vi "Dashboard Main.vi"() -> ()   [LabVIEW 2012]
uses:
  <vilib>/event_ctls.llb/eventvkey.ctl
  <vilib>/Utility/config.llb/Read Key (String).vi
  <vilib>/Utility/config.llb/Read Key (I32).vi
  <vilib>/Utility/config.llb/Write Key (String).vi
  <vilib>/Utility/config.llb/Write Key (I32).vi
  <vilib>/Utility/config.llb/NI_LVConfig.lvlib
panel:
  out "Battery Value":dbl(slide) scale=0.0..14.0 scale format="%#_2e"
  out "Battery":sgl(graph)
  in  "Camera Settings":T1={"Frate Rate"=30, "Compression"=30, "Size"=0} {"Frate Rate" scale=1.0..30.0; "Size" items=["640x480", "320x240", "160x120"]}
  out "Mode":T2(ring)=enum.""
  out "Camera IP":string="10.16.76.11"
  out "JS1 Z":dbl(slide) scale=-1.0..1.0 scale format="%#_2e"
  out "JS2 Z":dbl(slide) scale=-1.0..1.0 scale format="%#_2e"
  out "Joystick 1":cluster{"X":dbl, "Y":dbl}[](graph)
  out "Joystick 2":cluster{"X":dbl, "Y":dbl}[](graph)
  out "JS Buttons 1":T3
  out "JS Buttons 2":T3
  out "MotorSlide4":dbl(slide) scale=-1.0..1.0 scale format="%#_2e"
  out "MotorSlide3":dbl(slide) scale=-1.0..1.0 scale format="%#_2e"
  out "MotorSlide2":dbl(slide) scale=-1.0..1.0 scale format="%#_2e"
  in  "MotorName3":string="Front Left"
  in  "MotorName4":string="Front Right"
  in  "MotorName1":string="Rear Left"
  in  "MotorName2":string="Rear Right"
  out "MotorChart4":dbl(graph)
  out "MotorChart3":dbl(graph)
  out "MotorChart2":dbl(graph)
  out "MotorSlide1":dbl(slide) scale=-1.0..1.0 scale format="%#_2e"
  out "MotorChart1":dbl(graph)
  out "Robot IP":string="0.0.0.0"
  in  "Dashboard Tab":enum32{"Operation", "Test", "Checklist"}(tab)
  in  "Checkbox 2":bool
  in  "Checkbox 1":bool
  in  "Slider 1":dbl(slide) scale=0.0..100.0
  in  "Slider":dbl(slide) scale=0.0..100.0 scale format="%#_3g"
  in  "On/Off":bool caption="Solenoid"
  in  "Test Name":u16(ring) items=["Select the test to run...", "Example Test", "-------------------------------", "List of tests is built in robot code.", "Replace with your own automated tests."]
  in  "Test Tree":string(tree)
  in  "Motor":cluster{"Value":dbl, "Enable":bool} {"Value" scale=-1.0..1.0 scale format="%#_3g"}
  out "Progress":T4 {"Test Progress" scale=0.0..100.0}
  in  "Rev/Fwd":cluster{"Forward":bool, "Reverse":bool}
  in  "Ring":u16(ring) items=["Auto", "Fixed indoor", "Fixed outdoor 1", "Fixed outdoor 2", "Fixed fluorescent 1", "Fixed fluorescent 2", "Hold current"]
  in  "Listbox":i32(listbox)
  in  "Viewer":T5(tab)
  out "Mbps":dbl format="%#.1g"
  in  "Enable":bool=TRUE
  in  "DB Camera Config":bool
  out "Mbps":bool
  out "fps":dbl format="%#.1g"
  out "Image Error Message":string="Timeout in Camera Communications"
  out "Camera Image":T6(plugin-control)
  out "Buttons 1":cluster{"1":bool, "2":bool, "3":bool}
  out "Kinect 1":cluster{"X":dbl, "Y":dbl, "Z":dbl} {"X" scale=1.0..-1.0; "Y" scale=1.0..-1.0; "Z" scale=1.0..-1.0}
  out "Buttons 2":cluster{"1":bool, "2":bool, "3":bool}
  out "Kinect 2":cluster{"X":dbl, "Y":dbl, "Z":dbl} {"X" scale=1.0..-1.0; "Y" scale=1.0..-1.0; "Z" scale=1.0..-1.0}
  out "Version":string
  out "Skeleton Picture":picture
  out "Players":i8
  out "Tree":string(tree)
  # "Drive & Motors"
  # "Robot IP:"
  # "Customize by placing controls and indicators here and name to match\nDashboard Variables on robot."
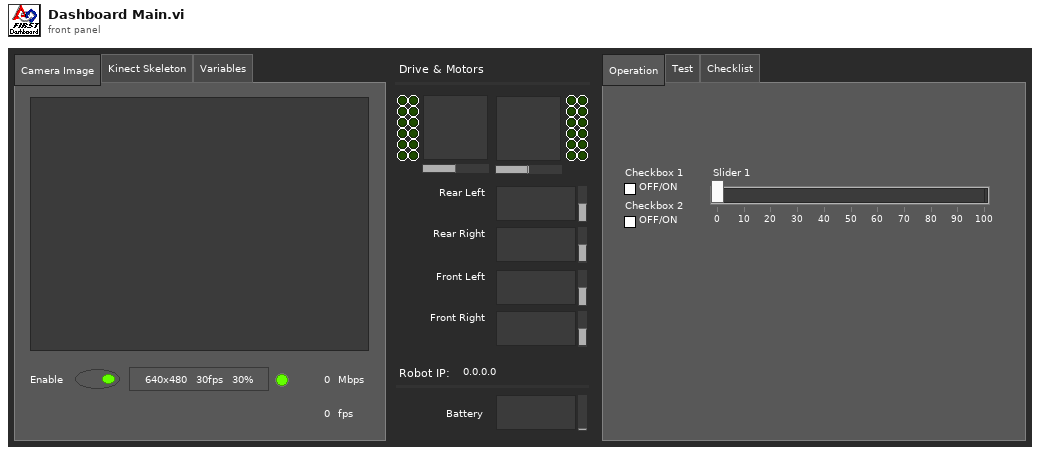
[diagram p1: front panel]
types:
  T1 = cluster{"Frate Rate":i32, "Compression":i32, "Size":u16}
  T2 = enum8{"Tele-Op Disabled", "Tele-Op Enabled", "Auto Disabled", "Auto Enabled", "Test Disabled", "Test Enabled", ""}
  T3 = cluster{bool, bool, bool, bool, bool, bool, bool, bool, bool, bool, bool, bool}
  T4 = cluster{"Test Progress":u8, "Test Progress Text":string}
  T5 = enum32{"Camera Image", "Kinect Skeleton", "Variables"}
  T6 = typedef "IMAQ Image.ctl" = refnum<image>
  T7 = typedef "Image Type" = u32
  T8 = cluster{"Competition mode":bool, "Robot Link":bool, "Autonomous":bool, "Enabled":bool, "E-Stop":bool, "Simulated":bool, "TestMode":bool, "Docked Window":bool}
  T9 = cluster{"Boolean Array[0]":bool, "Boolean Array[1]":bool, "Boolean Array[2]":bool, "Boolean Array[3]":bool, "Boolean Array[4]":bool, "Boolean Array[5]":bool, "Boolean Array[6]":bool, "Boolean Array[7]":bool, "Boolean Array[8]":bool, "Boolean Array[9]":bool, "Boolean Array[10]":bool, "Boolean Array[11]":bool}
  T10 = typedef "LVBoundsTypeDef.ctl" = cluster{"Width":u32, "Height":u32}
  T11 = typedef "SkeletonTrackState.ctl" = enum32{"NotTracked", "PositionOnly", "Tracked"}
  T12 = cluster{"TrackingState":u8[], "Position":cluster{"x":sgl, "y":sgl, "z":sgl}, cluster{"x":sgl, "y":sgl, "z":sgl, sgl}[], "TrackState":T11}
  T13 = cluster{cluster{"ScaledToPercentRange":dbl, "ScaledToPercentRange":dbl, "ScaledToPercentRange":dbl}, cluster{bool, bool, bool}}[]
  T14 = cluster{cluster{"ScaledToPercentRange":dbl, "ScaledToPercentRange":dbl, "ScaledToPercentRange":dbl}, cluster{bool, bool, bool}}
  T15 = cluster{"ScaledToPercentRange":dbl, "ScaledToPercentRange":dbl, "ScaledToPercentRange":dbl}
  T16 = typedef "LVRectTypeDef.ctl" = cluster{"Left":i16, "Top":i16, "Right":i16, "Bottom":i16}
  T17 = typedef "NI_LVConfig.lvlib/Config Data RefNum.ctl" = refnum<k1>
  T18 = typedef "eventvkey.ctl" = enum16{"ASCII", "Enter", "Return", "Shift", "Ctrl", "Alt", "Cmd", "Opt", "Caps", "NumLock", "Clear", "Break", "Up", "Down", "Left", "Right", "Insert", "Delete", "Home", "End", "PageUp", "PageDown", "Escape", "Help", "Pause", "ScrollLock", "F1", "F2", "F3", "F4", "F5", "F6", "F7", "F8", "F9", "F10", "F11", "F12", "F13", "F14", "F15", "F16", "F17", "F18", "F19", "F20", "F21", "F22", "F23", "F24", "Play", "VolumeUp", "VolumeDown", "Mute", "Two Byte Char"}
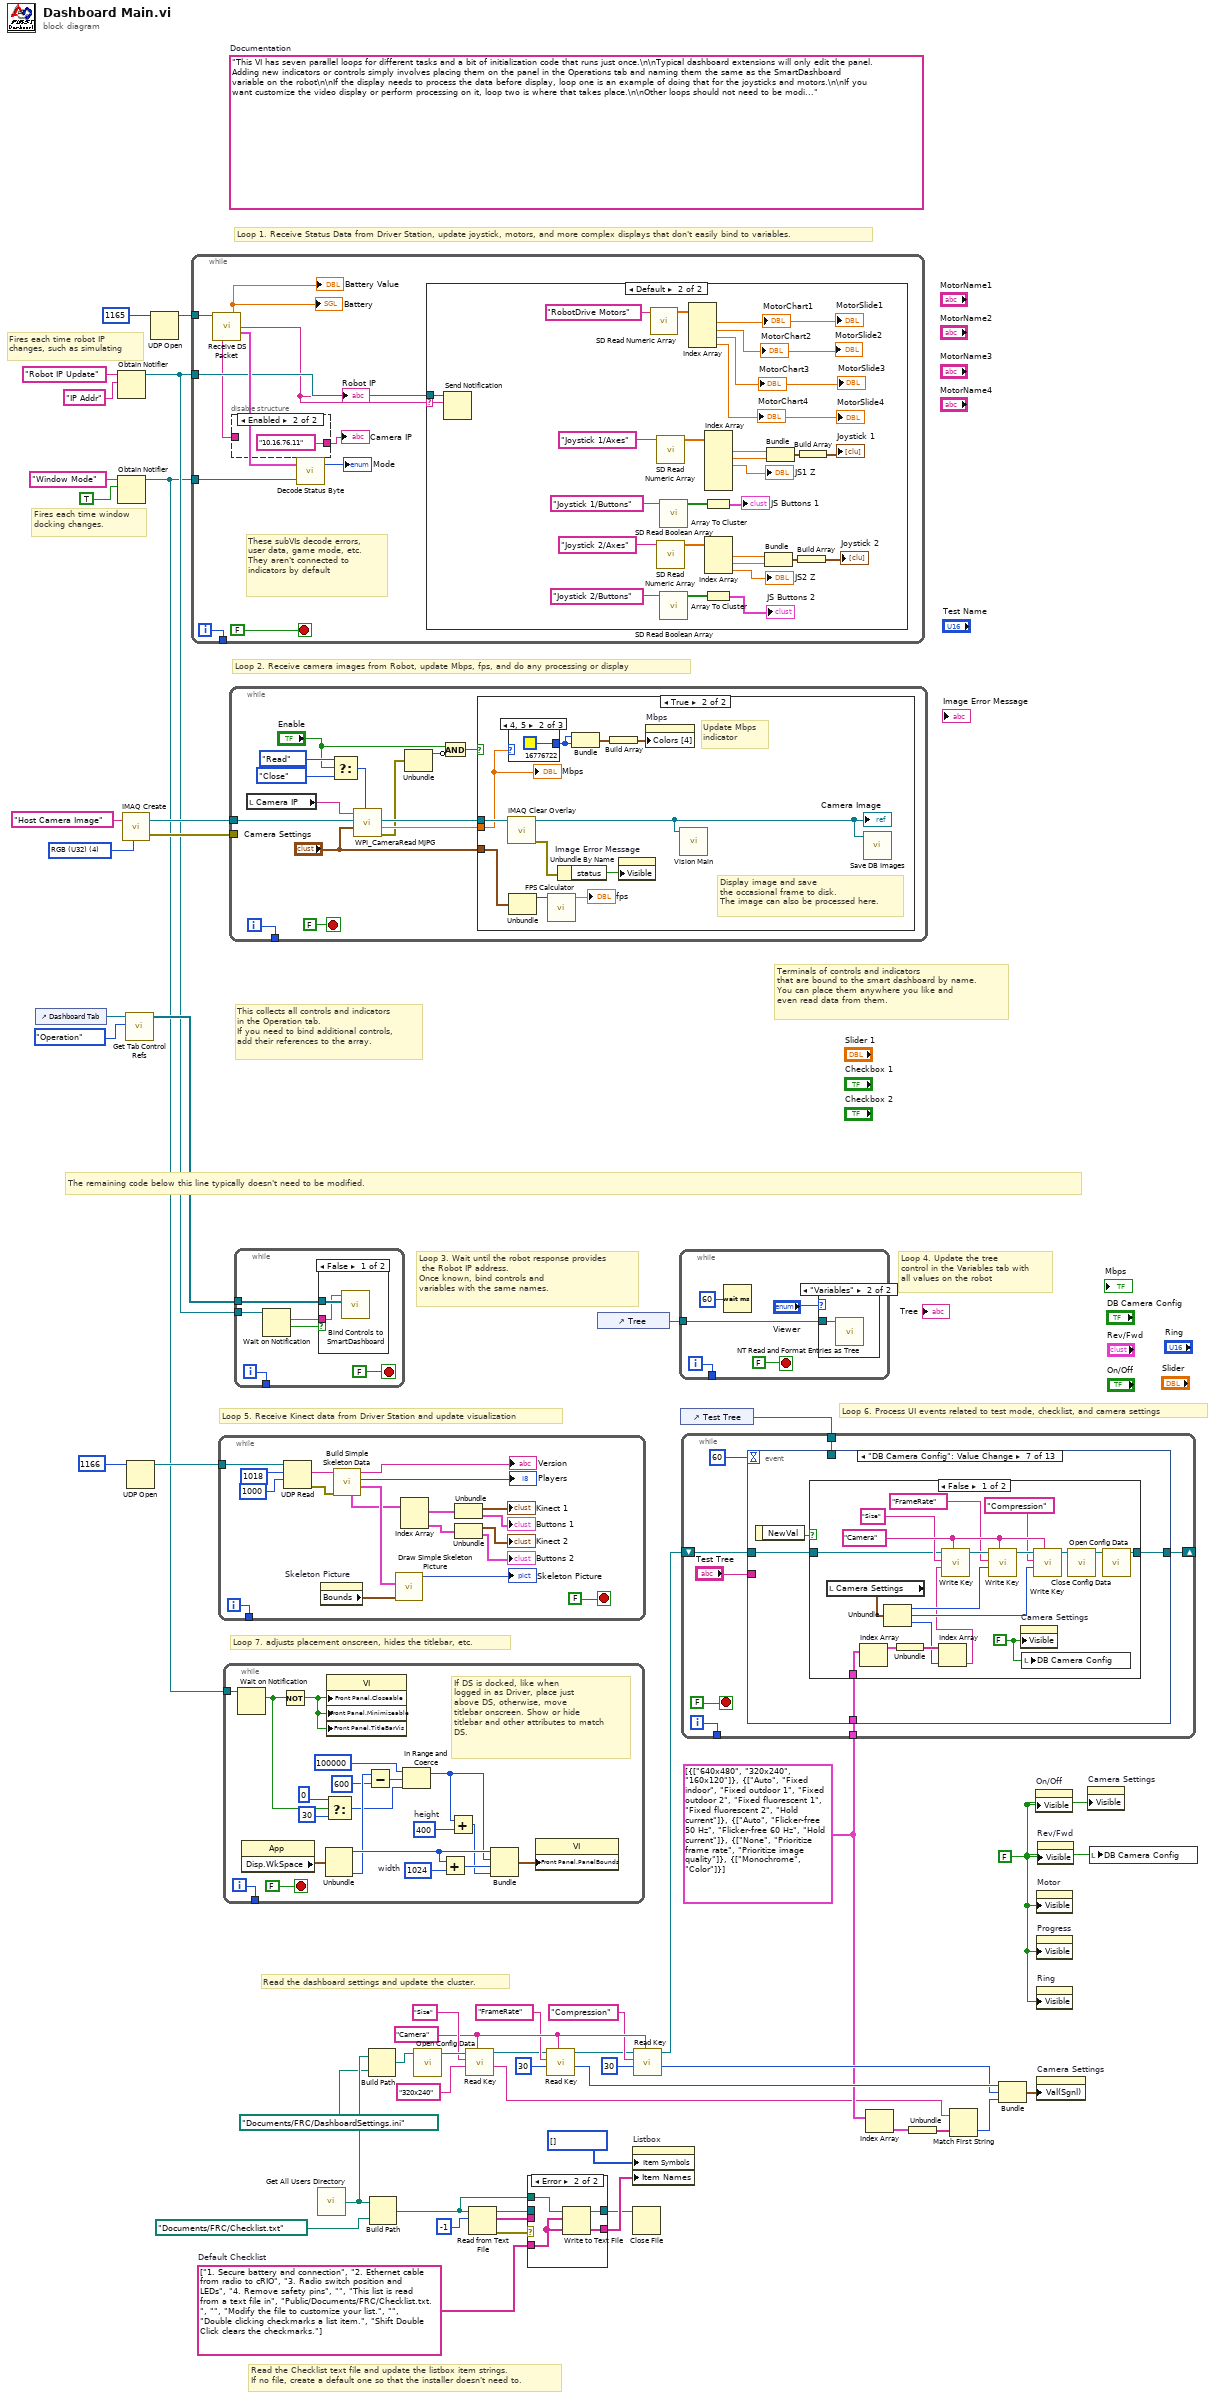
[diagram p0: block diagram]
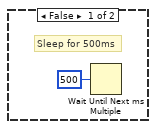
[diagram p3: hidden frame]
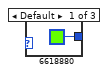
[diagram p4: hidden frame]
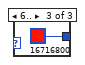
[diagram p5: hidden frame]
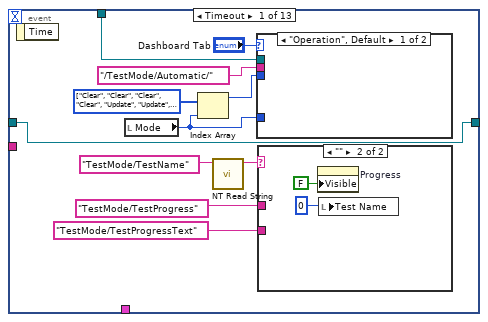
[diagram p7: hidden frame]
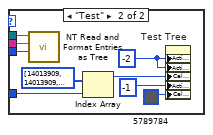
[diagram p8: hidden frame]
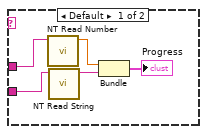
[diagram p9: hidden frame]
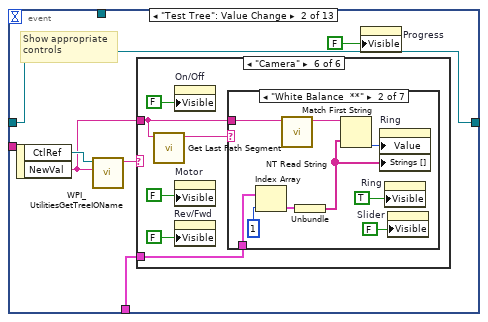
[diagram p10: hidden frame]
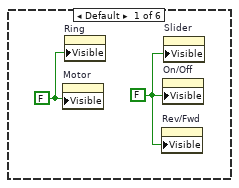
[diagram p11: hidden frame]
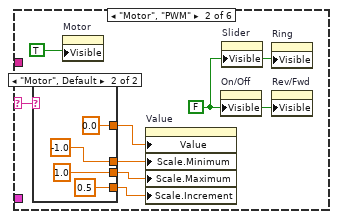
[diagram p12: hidden frame]
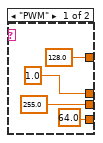
[diagram p13: hidden frame]
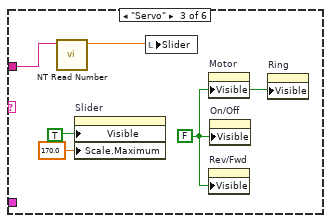
[diagram p14: hidden frame]
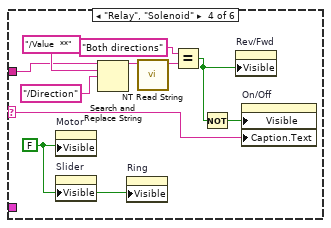
[diagram p15: hidden frame]
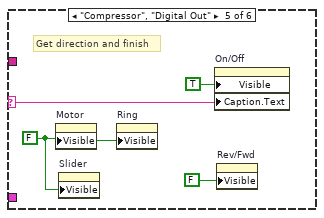
[diagram p16: hidden frame]
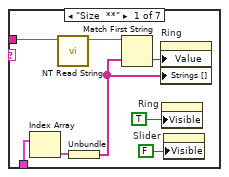
[diagram p17: hidden frame]
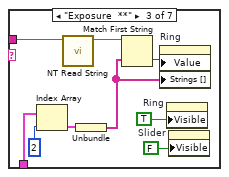
[diagram p18: hidden frame]
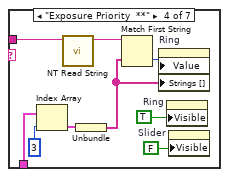
[diagram p19: hidden frame]
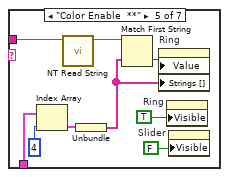
[diagram p20: hidden frame]
diagram:
  w21 = "Camera"
  w13 = cluster{string[]}[] [{["640x480", "320x240", "160x120"]}, {["Auto", "Fixed indoor", "Fixed outdoor 1", "Fixed outdoor 2", "Fixed fluorescent 1", "Fixed fluorescent 2", "Hold current"]}, {["Auto", "Flicker-free 50 Hz", "Flicker-free 60 Hz", "Hold current"]}, {["None", "Prioritize frame rate", "Prioritize image quality"]}, {["Monochrome", "Color"]}]
  w29 = string[] ["1. Secure battery and connection", "2. Ethernet cable from radio to cRIO", "3. Radio switch position and LEDs", "4. Remove safety pins", "", "This list is read from a text file in", "Public/Documents/FRC/Checklist.txt.", "", "Modify the file to customize your list.", "", "Double clicking checkmarks a list item.", "Shift Double Click clears the checkmarks."]  # Default Checklist
  w27 = FALSE ("Visible")
  (unwired) "This VI has seven parallel loops for different tasks and a bit of initialization code that runs just once.\n\nTypical dashboard extensions will only edit the panel. Adding new indicators or controls simply involves placing them on the panel in the Operations tab and naming them the same as the SmartDashboard variable on the robot\n\nIf the display needs to process the data before display, loop one is an example of doing that for the joysticks and motors.\n\nIf you want customize the video display or perform processing on it, loop two is where that takes place.\n\nOther loops should not need to be modified. They are pretty standard, and document the task they perform."  # Documentation
  w50 = T7 4 items=["Grayscale (U8)", "Grayscale (I16)", "Grayscale (SGL)", "Complex (CSG)", "RGB (U32)", "HSL (U32)", "RGB (U64)"] ("Image Type")
  # "Fires each time robot IP\nchanges, such as simulating"
  # "Fires each time window\ndocking changes."
  # "Read the Checklist text file and update the listbox item strings.\nIf no file, create a default one so that the installer doesn't need to."
  # "This collects all controls and indicators\nin the Operation tab.\nIf you need to bind additional controls,\nadd their references to the array."
  # "The remaining code below this line typically doesn't need to be modified."
  # "Loop 6. Process UI events related to test mode, checklist, and camera settings"
  # "Read the dashboard settings and update the cluster."
  # "Terminals of controls and indicators\nthat are bound to the smart dashboard by name.\nYou can place them anywhere you like and\neven read data from them."
  # "Loop 4. Update the tree\ncontrol in the Variables tab with\nall values on the robot"
  # "Loop 3. Wait until the robot response provides\n the Robot IP address.\nOnce known, bind controls and\nvariables with the same names."
  # "Loop 5. Receive Kinect data from Driver Station and update visualization"
  # "Loop 7. adjusts placement onscreen, hides the titlebar, etc."
  # "Loop 1. Receive Status Data from Driver Station, update joystick, motors, and more complex displays that don't easily bind to variables."
  # "Loop 2. Receive camera images from Robot, update Mbps, fps, and do any processing or display"
  n1 = control-ref of="Dashboard Tab"() -> (w43:refnum<vi>)
  n2 = Obtain Notifier(name (unnamed)="Robot IP Update", notification data type="IP Addr" ("name (unnamed)")) -> (notifier out=w40:refnum<notifier>)  [unwired: 2 in, 2 out]
  n3 = Obtain Notifier(name (unnamed)="Window Mode", notification data type=TRUE) -> (notifier out=w33:refnum<notifier>)  [unwired: 2 in, 2 out]
  n4 = call "IMAQ Create"("Image Name"="Host Camera Image", "Image Type"=w50) -> ("New Image"=w48:T6, "error out"=w47:errorcluster)  [unwired: 2 in, 1 out]
  n5 = call <vilib>:"Get Tab Control Refs.vi"("Page Index"=enum32{"Operation", "Test"}."Operation" ("Dashboard Tab"), "TabControl in"=w43) -> ("ControlsOnPage"=w44:refnum<vi>[])  [unwired: 9 in]
  n6 = UDP Open(11:u16 1166 ("port")) -> (port=w45:refnum<k16>)  [unwired: 2 in, 4 out]
  n7 = UDP Open(11:u16 1165 ("port")) -> (port=w51:refnum<k16>)  [unwired: 2 in, 4 out]
  n8 = while {
    tunnel: w51 -> [w61]
    tunnel: w40 -> [w56]
    tunnel: w33 -> [w59]
    tunnel: [w57] -> _
    i -> [w57]
    stop <- FALSE stop-if-true
    # "These subVIs decode errors, user data, game mode, etc.\nThey aren't connected to indicators by default"
    n9 = call "Receive DS Packet.vi"("Recv Socket"=w61) -> ("Battery"=→"Battery" →"Battery Value":sgl, "Robot IP Address"=w55:string, "Status"=w62:T8, "Camera IP Address"=w53:string)  [unwired: 1 in, 10 out]
    "Robot IP" <- w55
    n10 = disable-structure shown="Enabled" {
      disable-tunnel: [w64 "10.16.76.11" ("Camera IP")] -> w54
      disable-tunnel: w53 -> [w64 _]
      frame Disabled {
      }
      frame Enabled {
      }
    }
    "Camera IP" <- w54
    n11 = call "Decode Status Byte.vi"("Window Mode Notifier"=w59, "Status"=w62) -> ("Mode"=→"Mode":T2)  [unwired: 1 out]
    n12 = case shown="Default" w55 {
      selector: w55 -> [_ w66]
      tunnel: w56 -> [_ w67]
      frame "0.0.0.0" {
        # "Robot not responding, don't poll the variables"
      }
      frame Default {
        n13 = Send Notification(notification=w66, notifier=w67) -> ()  [unwired: 1 in, 2 out]
        n14 = call <vilib>:"SD Read Numeric Array.vi"("Name"="RobotDrive Motors") -> ("Numeric Array"=w90:dbl[])  [unwired: 8 in, 2 out]
        n15 = call <vilib>:"SD Read Numeric Array.vi"("Name"="Joystick 1/Axes") -> ("Numeric Array"=w83:dbl[])  [unwired: 8 in, 2 out]
        n16 = call <vilib>:"SD Read Numeric Array.vi"("Name"="Joystick 2/Axes") -> ("Numeric Array"=w77:dbl[])  [unwired: 8 in, 2 out]
        n17 = call <vilib>:"SD Read Boolean Array.vi"("Name"="Joystick 1/Buttons") -> ("Boolean Array"=w85:bool[])  [unwired: 8 in, 2 out]
        n18 = call <vilib>:"SD Read Boolean Array.vi"("Name"="Joystick 2/Buttons") -> ("Boolean Array"=w76:bool[])  [unwired: 8 in, 2 out]
        n19 = Index Array(array=w90) -> (element #1=→"MotorChart1" →"MotorSlide1":dbl, element #2=→"MotorSlide2" →"MotorChart2":dbl, element #3=→"MotorChart3" →"MotorSlide3":dbl, element #4=→"MotorChart4" →"MotorSlide4":dbl)  [unwired: 4 in]
        n20 = Array To Cluster(array=w85) -> (cluster=→"JS Buttons 1":T9)
        n21 = Array To Cluster(array=w76) -> (cluster=→"JS Buttons 2":T9)
        n22 = Index Array(array=w83) -> (element #1=w80:dbl, element #2=w81:dbl, element #3=→"JS1 Z":dbl)  [unwired: 6 in, 3 out]
        n23 = Index Array(array=w77) -> (element #1=w72:dbl, element #2=w71:dbl, element #3=→"JS2 Z":dbl)  [unwired: 3 in]
        n24 = Bundle("Numeric"=w72, "Numeric"=w71) -> (w73:cluster{"Numeric":dbl, "Numeric":dbl})  [unwired: 1 in]
        n25 = Bundle("Numeric"=w80, "Numeric"=w81) -> (w79:cluster{"Numeric":dbl, "Numeric":dbl})  [unwired: 1 in]
        n26 = Build Array(w73) -> (→"Joystick 2":cluster{"Numeric":dbl, "Numeric":dbl}[])
        n27 = Build Array(w79) -> (→"Joystick 1":cluster{"Numeric":dbl, "Numeric":dbl}[])
      }
    }
  }
  n28 = while {
    tunnel: w45 -> [w110]
    tunnel: [w95] -> _
    i -> [w95]
    stop <- FALSE stop-if-true
    n29 = UDP Read(connection ID=w110, max size (548)=1018 ("bytes to read"), timeout ms (25000)=1000) -> (data out=w104:string, error out=w94:errorcluster)  [unwired: 1 in, 3 out]
    n30 = property on="Skeleton Picture" class="Pict"() -> ("Bounds"=w106:T10)  [unwired: 2 in, 2 out]
    n31 = call "Build Simple Skeleton Data.vi"("error in (no error)"=w94, "data in"=w104) -> ("Skeleton Data"=w105:T12, "NumPlayers"=→"Players":i8, "Version String"=→"Version":string, "Simple Joystick Info"=w102:T13)  [unwired: 5 in, 1 out]
    n32 = call "Draw Simple Skeleton Picture.vi"("Bounds"=w106, "Simple Skeleton"=w105) -> ("new picture out"=→"Skeleton Picture":picture)  [unwired: 9 in]
    n33 = Index Array(array=w102) -> (element #1=w101:T14, element #2=w100:T14)  [unwired: 2 in]
    n34 = Unbundle(w101) -> (→"Kinect 1":T15, →"Buttons 1":cluster{bool, bool, bool})
    n35 = Unbundle(w100) -> (→"Kinect 2":T15, →"Buttons 2":cluster{bool, bool, bool})
  }
  n36 = while {
    tunnel: w33 -> [w131]
    tunnel: [w129] -> _
    i -> [w129]
    stop <- FALSE stop-if-true
    w121 = 1024  # width
    w124 = 400  # height
    # "If DS is docked, like when\nlogged in as Driver, place just\nabove DS, otherwise, move\ntitlebar onscreen. Show or hide\ntitlebar and other attributes to match\nDS."
    n37 = Wait on Notification(notifier=w131) -> (notification=w116:bool)  [unwired: 3 in, 3 out]
    n38 = property class="App"() -> ("Disp.WkSpace"=w127:T16)  [unwired: 2 in, 2 out]
    n39 = Not(x=w116) -> (.not. x?=w130:bool)
    n40 = Unbundle(w127) -> ("Left"=w125:i16, "Bottom"=w122:i16)  [unwired: 2 out]
    n41 = Select(t=0, s=w116, f=30) -> (s? t:f=w115:i32)
    n42 = property class="VI"("Front Panel.Closeable"=w130, "Front Panel.Minimizeable"=w130, "Front Panel.TitleBarVis"=w130) -> ()  [unwired: 2 in, 2 out]
    n43 = Subtract(x=w122, y=600) -> (x-y=w119:i32)
    n44 = In Range and Coerce(upper limit=100000, x=w119, lower limit=w115) -> (coerced(x)=w113:i32)  [unwired: 1 out]
    n45 = Add(x=w125, y=w121) -> (x+y=w126:i32)
    n46 = Add(x=w113, y=w124) -> (x+y=w123:i32)
    n47 = Bundle("Left"=w125, w113, w126, w123) -> (w128:cluster{"Left":i16, i32, i32, i32})  [unwired: 1 out]
    n48 = property class="VI"("Front Panel.PanelBounds"=w128) -> ()  [unwired: 2 in, 2 out]
  }
  n49 = while {
    tunnel: w48 -> [w142]
    tunnel: w47 -> [_]
    tunnel: [w145] -> _
    i -> [w145]
    stop <- FALSE stop-if-true
    n50 = local read "Camera IP"() -> (w144:string)
    n51 = Select(t=enum16{"Read", "Reopen", "Close"}."Read" ("Operation"), s="Enable", f=enum16{"Read", "Reopen", "Close"}."Close" ("Operation")) -> (s? t:f=w137:enum16{"Read", "Reopen", "Close"})
    n52 = call <vilib>:"WPI_CameraRead MJPG.vi"("Operation"=w137, "Camera Settings"="Camera Settings", "Image"=w142, "address"=w144) -> ("error out"=w136:errorcluster, "Bandwidth (kbps)"=w140:dbl, "Image Out"=w141:T6)  [unwired: 5 in]
    n53 = Unbundle(w136) -> ("status"=w134:bool)  [unwired: 2 out]
    n54 = Compound Arithmetic op=AND("Enable", invert w134) -> (w133:bool)
    n55 = case shown="True" w133 {
      tunnel: "Camera Settings" -> [_ w150]
      tunnel: w141 -> [_ w153]
      tunnel: w140 -> [_ w152]
      frame False {
        # "Sleep for 500ms"
        n56 = Wait Until Next ms Multiple(millisecond multiple=u32 500) -> ()  [unwired: 1 out]
      }
      frame True {
        # "Display image and save\nthe occasional frame to disk.\nThe image can also be processed here."
        # "Update Mbps\nindicator"
        n57 = call "IMAQ Clear Overlay"("Image"=w153) -> ("error out"=w157:errorcluster, "Image Out"=w148:T6)  [unwired: 2 in, 7 out]
        "Camera Image" <- w148
        n58 = case shown="4, 5" w152 {
          tunnel: [u32 6618880 ("Color Box") u32 16776722 ("Color Box") u32 16716800 ("Color Box")] -> w154
          frame Default {
          }
          frame 4, 5 {
          }
          frame 6.. {
          }
        }
        n59 = Unbundle(w150) -> ("Frate Rate"=w149:i32)  [unwired: 2 out]
        n60 = call "FPS Calculator.vi"("Average Count"=w149) -> ("fps"=→"fps":dbl)  [unwired: 10 in]
        n61 = Unbundle By Name(w157) -> ("status"=w158:bool)
        n62 = Bundle("Color Box"=w154, "Color Box"=w154) -> (w156:cluster{"Color Box":u32, "Color Box":u32})  [unwired: 1 out]
        n63 = Build Array(w156) -> (w155:cluster{"Color Box":u32, "Color Box":u32}[])
        n64 = property on="Image Error Message" class="Str"("Visible"=w158) -> ()  [unwired: 2 in, 2 out]
        n65 = property on="Mbps" class="Bool (strict)"("Colors [4]"=w155) -> ()  [unwired: 2 in, 2 out]
        n66 = call "Vision Main.vi"("Camera Image"=w148) -> ()  [unwired: 11 in]
        n67 = call "Save DB Images.vi"("Image"=w148) -> ()  [unwired: 2 in, 1 out]
        "Mbps" <- w152
      }
    }
  }
  n68 = while {
    tunnel: w44 -> [w167]
    tunnel: w40 -> [w164]
    tunnel: [w162] -> _
    i -> [w162]
    stop <- FALSE stop-if-true
    n69 = Wait on Notification(notifier=w164) -> (notification=w163:string, timed out?=w165:bool)  [unwired: 3 in, 2 out]
    n70 = case shown="False" w165 {
      tunnel: w167 -> [w169 _]
      tunnel: w163 -> [w168 _]
      frame False {
        n71 = call <vilib>:"Bind Controls to SmartDashboard.vi"("Bound Control Refs"=w169, "Server IP Address"=w168) -> ()  [unwired: 10 in]
      }
      frame True {
      }
    }
  }
  n72 = call "Get All Users Directory.vi"() -> ("All User Path"=w26:path)
  n73 = Build Path(base path=w26, name or relative path=path "Documents/FRC/DashboardSettings.ini") -> (appended path=w25:path)
  n74 = Build Path(base path=w26, name or relative path=path "Documents/FRC/Checklist.txt") -> (appended path=w30:path)
  n75 = call <vilib>:"Open Config Data.vi"("configuration file path"=w25) -> ("refnum"=w24:T17)  [unwired: 8 in, 2 out]
  n76 = call-poly <vilib>:"Read Key.vi"("section"=w21, "default value"="320x240", "key"="Size", "refnum"=w24) -> ("value"=w11:string, "refnum out"=w6:T17)  [unwired: 2 in, 4 out]
  n77 = Read from Text File(file (use dialog)=w30, count=-1 ("timeout ms (25000)")) -> (refnum out=w8:refnum<file>, text=w31:string[], error out=w32:errorcluster)  [unwired: 2 in, 1 out]
  n78 = case shown="Error" w32 {
    tunnel: w31 -> [w171 _]
    tunnel: [w171 w173] -> w28
    tunnel: w29 -> [_ w173]
    tunnel: w30 -> [_ w174]
    tunnel: [w170 w172] -> w7
    tunnel: w8 -> [w170 _]
    frame No Error {
    }
    frame Error {
      n79 = Write to Text File(file (use dialog)=w174, text=w173) -> (refnum out=w172:refnum<file>)  [unwired: 2 in, 2 out]
    }
  }
  n80 = call-poly <vilib>:"Read Key.vi"("section"=w21, "default value"=30, "key"="FrameRate", "refnum"=w6) -> ("value"=w16:i32, "refnum out"=w5:T17)  [unwired: 1 in, 5 out]
  n81 = control-ref of="Tree"() -> (w2:refnum<vi>)
  n82 = property on="Listbox" class="LstBox (strict)"("Item Symbols"=i32[] [], "Item Names"=w28) -> ()  [unwired: 2 in, 2 out]
  n83 = Close File(refnum=w7) -> ()  [unwired: 1 in, 2 out]
  n84 = call-poly <vilib>:"Read Key.vi"("section"=w21, "default value"=30, "key"="Compression", "refnum"=w5) -> ("value"=w15:i32, "refnum out"=w3:T17)  [unwired: 1 in, 5 out]
  n85 = while {
    tunnel: [w176] -> _
    tunnel: w2 -> [w175]
    i -> [w176]
    stop <- FALSE stop-if-true
    n86 = Wait (ms)(milliseconds to wait=u32 60) -> ()  [unwired: 1 out]
    n87 = case shown="\"Variables\"" "Viewer" {
      tunnel: w175 -> [_ w180]
      frame Default {
      }
      frame "Variables" {
        n88 = call <vilib>:"NT Read and Format Entries as Tree.vi"("Tree Refnum"=w180) -> ()  [unwired: 9 in, 2 out]
      }
    }
  }
  n89 = control-ref of="Test Tree"() -> (w1:refnum<vi>)
  n90 = while {
    tunnel: w13 -> [w185]
    shift-right: [w184] -> _
    shift-left: w3 -> [w183]
    tunnel: [w182] -> _
    tunnel: w1 -> [w181]
    i -> [w182]
    stop <- FALSE stop-if-true
    n91 = event shown="[6] \"DB Camera Config\": Value Change" {
      selector: _ -> [_ _ _ _ _ _ _ _ _ _ _ _ _]
      dyn-events: _ -> [_ _ _ _ _ _ _ _ _ _ _ _ _]
      timeout: u32 60 ("milliseconds to wait") -> [_ _ _ _ _ _ _ _ _ _ _ _ _]
      tunnel: w181 -> [w195 _ _ _ _ _ _ _ _ _ _ _ _]
      tunnel: "Test Tree" -> [_ _ _ _ _ _ _ _ w389 w397 w399 w403 w411]
      tunnel: w185 -> [_ w217 _ _ _ _ w353 w383 _ _ _ _ _]
      tunnel: [w189 w216 _ w319 w327 w339 w352 w376 w388 w395 w398 w402 w410] -> w184
      tunnel: w183 -> [w189 w216 _ w319 w327 w339 w351 w376 w388 w395 w398 w402 w410]
      event Timeout {
        w194 = enum16{"Update", "Clear"}[] [enum."Clear", enum."Clear", enum."Clear", enum."Clear", enum."Update", enum."Update", enum."Clear"] items=["Update", "Clear"]
        n92 = event-data() -> ()  [unwired: 1 in, 1 out]
        n93 = local read "Mode"() -> (w192:T2)
        n94 = Index Array(array=w194, index=w192) -> (element=w193:enum16{"Update", "Clear"})
        n95 = call <vilib>:"NT Read String.vi"("Name"="TestMode/TestName") -> ("String"=w198:string)  [unwired: 9 in, 1 out]
        n96 = case shown="\"Operation\", Default" "Dashboard Tab" {
          tunnel: w195 -> [_ w208]
          tunnel: "/TestMode/Automatic/" ("Name Pattern") -> [_ w207]
          tunnel: w193 -> [_ w206]
          tunnel: w192 -> [_ w204]
          frame "Operation", Default {
          }
          frame "Test" {
            w203 = -2 ("Active Item:Row Number")
            n97 = call <vilib>:"NT Read and Format Entries as Tree.vi"("Operation"=w206, "Name Pattern"=w207, "Tree Refnum"=w208) -> ()  [unwired: 7 in, 2 out]
            n98 = Index Array(array=u32[] [14013909, 14013909, 14013909, 14013909, 14013909, 16777215, 14013909], index=w204) -> (element=w202:u32)
            n99 = property on="Test Tree" class="Tree (strict)"("Active Item Row Number"=w203, "ActiveColNum"=w203, "CellBG"=w202, "Active Item Row Number"=-1 ("Active Item:Row Number"), "CellBG"=u32 5789784 ("Color Box")) -> ()  [unwired: 2 in, 2 out]
          }
        }
        n100 = case shown="\"\"" w198 {
          tunnel: "TestMode/TestProgress" ("Name") -> [w210 _]
          tunnel: "TestMode/TestProgressText" ("Name") -> [w209 _]
          frame Default {
            n101 = call <vilib>:"NT Read Number.vi"("Name"=w210) -> ("Numeric"=w211:dbl)  [unwired: 9 in, 1 out]
            n102 = call <vilib>:"NT Read String.vi"("Name"=w209) -> ("String"=w212:string)  [unwired: 9 in, 1 out]
            n103 = Bundle("Numeric"=w211, "String"=w212) -> (→"Progress":cluster{"Numeric":dbl, "String":string})  [unwired: 1 in]
          }
          frame "" {
            n104 = property on="Progress" class="Clust (strict)"("Visible"=FALSE) -> ()  [unwired: 2 in, 2 out]
            n105 = local write "Test Name"(u16 0) -> ()
          }
        }
      }
      event "Test Tree": Value Change {
        # "Show appropriate\ncontrols"
        n106 = event-data() -> ("CtlRef"=w220:refnum<vi>, "NewVal"=w218:string)  [unwired: 1 in]
        n107 = call <vilib>:"WPI_UtilitiesGetTreeIOName.vi"("NewVal"=w218, "TreeControl in"=w220) -> ("I/O Name"=w221:string)  [unwired: 9 in]
        n108 = case shown="\"Camera\"" w221 {
          selector: w221 -> [_ w228 _ w246 w255 _]
          tunnel: w218 -> [_ _ w243 w245 _ w262]
          tunnel: w217 -> [_ _ _ _ _ w261]
          frame Default {
            w223 = FALSE ("Visible")
            w222 = FALSE ("Visible")
            n109 = property on="Motor" class="Clust (strict)"("Visible"=w222) -> ()  [unwired: 2 in, 2 out]
            n110 = property on="Ring" class="Ring (strict)"("Visible"=w222) -> ()  [unwired: 2 in, 2 out]
            n111 = property on="Rev/Fwd" class="Clust (strict)"("Visible"=w223) -> ()  [unwired: 2 in, 2 out]
            n112 = property on="On/Off" class="Bool (strict)"("Visible"=w223) -> ()  [unwired: 2 in, 2 out]
            n113 = property on="Slider" class="Slide (strict)"("Visible"=w223) -> ()  [unwired: 2 in, 2 out]
          }
          frame "Motor", "PWM" {
            w229 = FALSE ("Visible")
            n114 = case shown="\"Motor\", Default" w228 {
              tunnel: [1.0 ("Value") -1.0 ("Value")] -> w227
              tunnel: [255.0 ("Value") 1.0 ("Value")] -> w226
              tunnel: [128.0 ("Value") 0.0 ("Value")] -> w225
              tunnel: [64.0 ("Value") 0.5 ("Value")] -> w224
              frame "PWM" {
              }
              frame "Motor", Default {
              }
            }
            n115 = property on="Motor" class="Clust (strict)"("Visible"=TRUE) -> ()  [unwired: 2 in, 2 out]
            n116 = property on="Value" class="Slide (strict)"("Value"=w225, "Scale.Minimum"=w227, "Scale.Maximum"=w226, "Scale.Increment"=w224) -> ()  [unwired: 2 in, 2 out]
            n117 = property on="On/Off" class="Bool (strict)"("Visible"=w229) -> ()  [unwired: 2 in, 2 out]
            n118 = property on="Slider" class="Slide (strict)"("Visible"=w229) -> ()  [unwired: 2 in, 2 out]
            n119 = property on="Ring" class="Ring (strict)"("Visible"=w229) -> ()  [unwired: 2 in, 2 out]
            n120 = property on="Rev/Fwd" class="Clust (strict)"("Visible"=w229) -> ()  [unwired: 2 in, 2 out]
          }
          frame "Servo" {
            w241 = FALSE ("Visible")
            n121 = call <vilib>:"NT Read Number.vi"("Name"=w243) -> ("Numeric"=w242:dbl)  [unwired: 9 in, 1 out]
            n122 = property on="Slider" class="Slide (strict)"("Visible"=TRUE, "Scale.Maximum"=170.0 ("Scale.Range:Maximum")) -> ()  [unwired: 2 in, 2 out]
            n123 = local write "Slider"(w242) -> ()
            n124 = property on="Motor" class="Clust (strict)"("Visible"=w241) -> ()  [unwired: 2 in, 2 out]
            n125 = property on="Rev/Fwd" class="Clust (strict)"("Visible"=w241) -> ()  [unwired: 2 in, 2 out]
            n126 = property on="On/Off" class="Bool (strict)"("Visible"=w241) -> ()  [unwired: 2 in, 2 out]
            n127 = property on="Ring" class="Ring (strict)"("Visible"=w241) -> ()  [unwired: 2 in, 2 out]
          }
          frame "Relay", "Solenoid" {
            w244 = FALSE ("Visible")
            n128 = property on="Motor" class="Clust (strict)"("Visible"=w244) -> ()  [unwired: 2 in, 2 out]
            n129 = property on="Slider" class="Slide (strict)"("Visible"=w244) -> ()  [unwired: 2 in, 2 out]
            n130 = Search and Replace String(input string=w245, search string="/Value  **", replace string="/Direction") -> (result string=w251:string)  [unwired: 5 in, 3 out]
            n131 = property on="Ring" class="Ring (strict)"("Visible"=w244) -> ()  [unwired: 2 in, 2 out]
            n132 = call <vilib>:"NT Read String.vi"("Name"=w251) -> ("String"=w249:string)  [unwired: 9 in, 1 out]
            n133 = Equal?(x="Both directions", y=w249) -> (x = y?=w247:bool)
            n134 = Not(x=w247) -> (.not. x?=w248:bool)
            n135 = property on="Rev/Fwd" class="Clust (strict)"("Visible"=w247) -> ()  [unwired: 2 in, 2 out]
            n136 = property on="On/Off" class="Bool (strict)"("Visible"=w248, "Caption.Text"=w246) -> ()  [unwired: 2 in, 2 out]
          }
          frame "Compressor", "Digital Out" {
            w254 = FALSE ("Visible")
            # "Get direction and finish"
            n137 = property on="Motor" class="Clust (strict)"("Visible"=w254) -> ()  [unwired: 2 in, 2 out]
            n138 = property on="Slider" class="Slide (strict)"("Visible"=w254) -> ()  [unwired: 2 in, 2 out]
            n139 = property on="Ring" class="Ring (strict)"("Visible"=w254) -> ()  [unwired: 2 in, 2 out]
            n140 = property on="On/Off" class="Bool (strict)"("Visible"=TRUE, "Caption.Text"=w255) -> ()  [unwired: 2 in, 2 out]
            n141 = property on="Rev/Fwd" class="Clust (strict)"("Visible"=FALSE) -> ()  [unwired: 2 in, 2 out]
          }
          frame "Camera" {
            n142 = call <vilib>:"Get Last Path Segment.vi"("String in"=w262) -> ("String out"=w263:string)  [unwired: 10 in]
            n143 = property on="On/Off" class="Bool (strict)"("Visible"=FALSE) -> ()  [unwired: 2 in, 2 out]
            n144 = property on="Motor" class="Clust (strict)"("Visible"=FALSE) -> ()  [unwired: 2 in, 2 out]
            n145 = property on="Rev/Fwd" class="Clust (strict)"("Visible"=FALSE) -> ()  [unwired: 2 in, 2 out]
            n146 = case shown="\"White Balance  **\"" w263 {
              tunnel: w262 -> [w269 w278 w287 w296 w305 _ w311]
              tunnel: w261 -> [w267 w275 w284 w293 w302 _ _]
              frame "Size  **" {
                n147 = Index Array(array=w267) -> (element=w266:cluster{string[]})  [unwired: 1 in]
                n148 = call <vilib>:"NT Read String.vi"("Name"=w269) -> ("String"=w268:string)  [unwired: 9 in, 1 out]
                n149 = Unbundle(w266) -> (w264:string[])
                n150 = Match First String(2:w264, 3:w268) -> (0:w265:i32)  [unwired: 1 out]
                n151 = property on="Ring" class="Ring (strict)"("Value"=w265, "Strings []"=w264) -> ()  [unwired: 2 in, 2 out]
                n152 = property on="Ring" class="Ring (strict)"("Visible"=TRUE) -> ()  [unwired: 2 in, 2 out]
                n153 = property on="Slider" class="Slide (strict)"("Visible"=FALSE) -> ()  [unwired: 2 in, 2 out]
              }
              frame "White Balance  **" {
                n154 = Index Array(array=w275, index=1) -> (element=w276:cluster{string[]})
                n155 = call <vilib>:"NT Read String.vi"("Name"=w278) -> ("String"=w277:string)  [unwired: 9 in, 1 out]
                n156 = Unbundle(w276) -> (w273:string[])
                n157 = Match First String(2:w273, 3:w277) -> (0:w272:i32)  [unwired: 1 out]
                n158 = property on="Ring" class="Ring (strict)"("Value"=w272, "Strings []"=w273) -> ()  [unwired: 2 in, 2 out]
                n159 = property on="Ring" class="Ring (strict)"("Visible"=TRUE) -> ()  [unwired: 2 in, 2 out]
                n160 = property on="Slider" class="Slide (strict)"("Visible"=FALSE) -> ()  [unwired: 2 in, 2 out]
              }
              frame "Exposure  **" {
                n161 = Index Array(array=w284, index=2) -> (element=w285:cluster{string[]})
                n162 = call <vilib>:"NT Read String.vi"("Name"=w287) -> ("String"=w286:string)  [unwired: 9 in, 1 out]
                n163 = Unbundle(w285) -> (w281:string[])
                n164 = Match First String(2:w281, 3:w286) -> (0:w282:i32)  [unwired: 1 out]
                n165 = property on="Ring" class="Ring (strict)"("Value"=w282, "Strings []"=w281) -> ()  [unwired: 2 in, 2 out]
                n166 = property on="Ring" class="Ring (strict)"("Visible"=TRUE) -> ()  [unwired: 2 in, 2 out]
                n167 = property on="Slider" class="Slide (strict)"("Visible"=FALSE) -> ()  [unwired: 2 in, 2 out]
              }
              frame "Exposure Priority  **" {
                n168 = Index Array(array=w293, index=3) -> (element=w294:cluster{string[]})
                n169 = call <vilib>:"NT Read String.vi"("Name"=w296) -> ("String"=w295:string)  [unwired: 9 in, 1 out]
                n170 = Unbundle(w294) -> (w290:string[])
                n171 = Match First String(2:w290, 3:w295) -> (0:w291:i32)  [unwired: 1 out]
                n172 = property on="Ring" class="Ring (strict)"("Value"=w291, "Strings []"=w290) -> ()  [unwired: 2 in, 2 out]
                n173 = property on="Ring" class="Ring (strict)"("Visible"=TRUE) -> ()  [unwired: 2 in, 2 out]
                n174 = property on="Slider" class="Slide (strict)"("Visible"=FALSE) -> ()  [unwired: 2 in, 2 out]
              }
              frame "Color Enable  **" {
                n175 = Index Array(array=w302, index=4) -> (element=w303:cluster{string[]})
                n176 = call <vilib>:"NT Read String.vi"("Name"=w305) -> ("String"=w304:string)  [unwired: 9 in, 1 out]
                n177 = Unbundle(w303) -> (w299:string[])
                n178 = Match First String(2:w299, 3:w304) -> (0:w300:i32)  [unwired: 1 out]
                n179 = property on="Ring" class="Ring (strict)"("Value"=w300, "Strings []"=w299) -> ()  [unwired: 2 in, 2 out]
                n180 = property on="Ring" class="Ring (strict)"("Visible"=TRUE) -> ()  [unwired: 2 in, 2 out]
                n181 = property on="Slider" class="Slide (strict)"("Visible"=FALSE) -> ()  [unwired: 2 in, 2 out]
              }
              frame Default {
                n182 = property on="Ring" class="Ring (strict)"("Visible"=FALSE) -> ()  [unwired: 2 in, 2 out]
                n183 = property on="Slider" class="Slide (strict)"("Visible"=FALSE) -> ()  [unwired: 2 in, 2 out]
              }
              frame "Brightness  **", "Color Level  **", "Compression  **", "FPS  **", "Sharpness  **" {
                n184 = call <vilib>:"NT Read Number.vi"("Name"=w311) -> ("Numeric"=w310:dbl)  [unwired: 9 in, 1 out]
                n185 = local write "Slider"(w310) -> ()
                n186 = property on="Slider" class="Slide (strict)"("Visible"=TRUE, "Scale.Maximum"=100.0 ("Scale.Range:Maximum")) -> ()  [unwired: 2 in, 2 out]
                n187 = property on="Ring" class="Ring (strict)"("Visible"=FALSE) -> ()  [unwired: 2 in, 2 out]
              }
            }
          }
        }
        n188 = property on="Progress" class="Clust (strict)"("Visible"=FALSE) -> ()  [unwired: 2 in, 2 out]
      }
      event "Test Name": Mouse Enter {
        # "Populate the ring with the list of tests"
        n189 = event-data() -> ()  [unwired: 1 in, 1 out]
        n190 = call <vilib>:"NT Read String Array.vi"("Name"="TestMode/TestList") -> ("String Array"=w318:string[])  [unwired: 9 in, 1 out]
        n191 = Build Array (concatenate)("Select the test to run...", w318) -> (w317:string[])
        n192 = property on="Test Name" class="Ring (strict)"("Strings []"=w317) -> ()  [unwired: 2 in, 2 out]
      }
      event "Test Name": Value Change {
        w320 = FALSE ("Visible")
        # "Tell the robot the test name to run"
        n193 = event-data() -> ("NewVal"=w324:u16)  [unwired: 1 in]
        n194 = property on="Test Name" class="Ring (strict)"() -> ("Strings []"=w325:string[])  [unwired: 2 in, 2 out]
        n195 = local write "Progress"(T4 {"Test Progress"=0, "Test Progress Text"=""} ("Progress")) -> ()
        n196 = Index Array(array=w325, index=w324) -> (element=w323:string)
        n197 = call <vilib>:"NT Write String.vi"("String"=w323, "Name"="TestMode/TestName") -> ()  [unwired: 9 in, 1 out]
        n198 = property on="Progress" class="Clust (strict)"("Visible"=TRUE) -> ()  [unwired: 2 in, 2 out]
        n199 = property on="Motor" class="Clust (strict)"("Visible"=w320) -> ()  [unwired: 2 in, 2 out]
        n200 = property on="Slider" class="Slide (strict)"("Visible"=w320) -> ()  [unwired: 2 in, 2 out]
        n201 = property on="On/Off" class="Bool (strict)"("Visible"=w320) -> ()  [unwired: 2 in, 2 out]
        n202 = property on="Rev/Fwd" class="Clust (strict)"("Visible"=w320) -> ()  [unwired: 2 in, 2 out]
        n203 = property on="Ring" class="Ring (strict)"("Visible"=w320) -> ()  [unwired: 2 in, 2 out]
      }
      event "Listbox": Double Click {
        n204 = event-data() -> ("PlatMods.Shift"=w328:bool, "Row"=w330:i32)  [unwired: 1 in]
        n205 = case shown="False" w328 {
          tunnel: w330 -> [w334 _]
          tunnel: 1 -> [w333 _]
          frame False {
            n206 = property on="Listbox" class="LstBox (strict)"() -> ("Item Symbols"=w332:i32[])  [unwired: 2 in, 2 out]
            n207 = Replace Array Subset(array=w332, new element=w333, index=w334) -> (w331:i32[])
            n208 = property on="Listbox" class="LstBox (strict)"("Item Symbols"=w331) -> ()  [unwired: 2 in, 2 out]
          }
          frame True {
            w335 = 0 ("Top Row")
            n209 = property on="Listbox" class="LstBox (strict)"() -> ("Number of Rows"=w337:u32)  [unwired: 2 in, 2 out]
            n210 = Initialize Array(0, w337) -> (w336:i32[])
            n211 = property on="Listbox" class="LstBox (strict)"("Top Row"=w335, "Value"=w335, "Item Symbols"=w336) -> ()  [unwired: 2 in, 2 out]
          }
        }
      }
      event "Listbox": Key Down {
        n212 = event-data() -> ("VKey"=w341:T18)  [unwired: 1 in]
        n213 = case shown="\"Left\", \"Right\"" w341 {
          selector: w341 -> [w346 _]
          tunnel: eventvkey."Left" ("VKey") -> [w344 _]
          frame "Left", "Right" {
            n214 = Equal?(x=w344, y=w346) -> (x = y?=w345:bool)
            n215 = Select(t=0, s=w345, f=1) -> (s? t:f=w347:i32)
            n216 = property on="Listbox" class="LstBox (strict)"() -> ("Item Symbols"=w350:i32[])  [unwired: 2 in, 2 out]
            n217 = Replace Array Subset(array=w350, new element=w347, index="Listbox") -> (w349:i32[])
            n218 = property on="Listbox" class="LstBox (strict)"("Item Symbols"=w349) -> ()  [unwired: 2 in, 2 out]
          }
          frame Default {
          }
        }
      }
      event "DB Camera Config": Value Change {
        n219 = event-data() -> ("NewVal"=w354:bool)  [unwired: 1 in]
        n220 = case shown="False" w354 {
          tunnel: w353 -> [w363 _]
          tunnel: [w356 w374] -> w352
          tunnel: w351 -> [w355 w374]
          frame False {
            w370 = "Camera"
            w373 = FALSE ("Visible")
            n221 = local read "Camera Settings"() -> (w362:T1)
            n222 = Index Array(array=w363) -> (element=w366:cluster{string[]})  [unwired: 1 in]
            n223 = Unbundle(w362) -> ("Frate Rate"=w361:i32, "Compression"=w360:i32, "Size"=w364:u16)
            n224 = Unbundle(w366) -> (w365:string[])
            n225 = Index Array(array=w365, index=w364) -> (element=w359:string)
            n226 = call-poly <vilib>:"Write Key.vi"("section"=w370, "value"=w359, "key"="Size", "refnum"=w355) -> ("refnum out"=w372:T17)  [unwired: 2 in, 5 out]
            n227 = call-poly <vilib>:"Write Key.vi"("section"=w370, "value"=w361, "key"="FrameRate", "refnum"=w372) -> ("refnum out"=w371:T17)  [unwired: 1 in, 6 out]
            n228 = property on="Camera Settings" class="Clust (strict)"("Visible"=w373) -> ()  [unwired: 2 in, 2 out]
            n229 = local write "DB Camera Config"(w373) -> ()
            n230 = call-poly <vilib>:"Write Key.vi"("section"=w370, "value"=w360, "key"="Compression", "refnum"=w371) -> ("refnum out"=w357:T17)  [unwired: 1 in, 6 out]
            n231 = call <vilib>:"Close Config Data.vi"("refnum"=w357) -> ("file path"=w358:path)  [unwired: 2 in, 8 out]
            n232 = call <vilib>:"Open Config Data.vi"("configuration file path"=w358) -> ("refnum"=w356:T17)  [unwired: 8 in, 2 out]
          }
          frame True {
            n233 = property on="Camera Settings" class="Clust (strict)"("Visible"=TRUE) -> ()  [unwired: 2 in, 2 out]
          }
        }
      }
      event "Camera Settings": Value Change {
        n234 = event-data() -> ("NewVal"=w387:T1)  [unwired: 1 in]
        n235 = Index Array(array=w383) -> (element=w382:cluster{string[]})  [unwired: 1 in]
        n236 = Unbundle(w387) -> ("Frate Rate"=w378:i32, "Compression"=w377:i32, "Size"=w380:u16)
        n237 = Unbundle(w382) -> (w381:string[])
        n238 = Index Array(array=w381, index=w380) -> (element=w379:string)
        n239 = Format Into String(format string="%s   %dfps   %d%%", w379, w378, w377) -> (resulting string=w384:string)  [unwired: 2 in, 1 out]
        n240 = Build Array(w384) -> (w385:string[])
        n241 = property on="DB Camera Config" class="Bool (strict)"("Strings [4]"=w385) -> ()  [unwired: 2 in, 2 out]
      }
      event "Motor.Enable": Value Change {
        n242 = event-data() -> ("NewVal"=w393:bool)  [unwired: 1 in]
        n243 = Unbundle("Motor") -> ("Value"=w392:dbl)  [unwired: 1 out]
        n244 = Select(t=w392, s=w393, f=0.0) -> (s? t:f=w390:dbl)
        n245 = call <vilib>:"NT Write Number.vi"("Numeric"=w390, "Name"=w389) -> ()  [unwired: 9 in, 1 out]
      }
      event "Slider": Value Change {
        n246 = event-data() -> ("NewVal"=w396:dbl)  [unwired: 1 in]
        n247 = call <vilib>:"NT Write Number.vi"("Numeric"=w396, "Name"=w397) -> ()  [unwired: 9 in, 1 out]
      }
      event "On/Off": Value Change {
        n248 = event-data() -> ("NewVal"=w401:bool)  [unwired: 1 in]
        n249 = Boolean To (0,1)(Boolean=w401) -> (0, 1=w400:i16)
        n250 = call <vilib>:"NT Write Number.vi"("Numeric"=w400, "Name"=w399) -> ()  [unwired: 9 in, 1 out]
      }
      event "Rev/Fwd": Value Change {
        n251 = event-data() -> ("NewVal.Forward"=w409:bool, "NewVal.Reverse"=w408:bool)  [unwired: 1 in]
        n252 = Boolean To (0,1)(Boolean=w409) -> (0, 1=w405:i16)
        n253 = Boolean To (0,1)(Boolean=w408) -> (0, 1=w407:i16)
        n254 = Negate(x=w407) -> (-x=w406:i16)
        n255 = Add(x=w405, y=w406) -> (x+y=w404:i16)
        n256 = call <vilib>:"NT Write Number.vi"("Numeric"=w404, "Name"=w403) -> ()  [unwired: 9 in, 1 out]
      }
      event "Ring": Value Change {
        n257 = event-data() -> ("NewVal"=w413:u16)  [unwired: 1 in]
        n258 = property on="Ring" class="Ring (strict)"() -> ("Strings []"=w414:string[])  [unwired: 2 in, 2 out]
        n259 = Index Array(array=w414, index=w413) -> (element=w412:string)
        n260 = call <vilib>:"NT Write String.vi"("String"=w412, "Name"=w411) -> ()  [unwired: 9 in, 1 out]
      }
    }
  }
  n261 = Index Array(array=w13) -> (element=w14:cluster{string[]})  [unwired: 1 in]
  n262 = Unbundle(w14) -> (w12:string[])
  n263 = Match First String(2:w12, 3:w11) -> (0:w10:i32)  [unwired: 1 out]
  n264 = Bundle("value"=w16, "value"=w15, "index"=w10) -> (w4:cluster{"value":i32, "value":i32, "index":i32})  [unwired: 1 out]
  n265 = property on="On/Off" class="Bool (strict)"("Visible"=w27) -> ()  [unwired: 2 in, 2 out]
  n266 = property on="Motor" class="Clust (strict)"("Visible"=w27) -> ()  [unwired: 2 in, 2 out]
  n267 = property on="Progress" class="Clust (strict)"("Visible"=w27) -> ()  [unwired: 2 in, 2 out]
  n268 = property on="Ring" class="Ring (strict)"("Visible"=w27) -> ()  [unwired: 2 in, 2 out]
  n269 = property on="Camera Settings" class="Clust (strict)"("Val(Sgnl)"=w4) -> ()  [unwired: 2 in, 2 out]
  n270 = property on="Rev/Fwd" class="Clust (strict)"("Visible"=w27) -> ()  [unwired: 2 in, 2 out]
  n271 = property on="Camera Settings" class="Clust (strict)"("Visible"=w27) -> ()  [unwired: 2 in, 2 out]
  n272 = local write "DB Camera Config"(w27) -> ()
